vi "Temp Cluster Build.vi"() -> (8 "Bus":T1)   [LabVIEW 2011]
uses:
  Controls/1553_Bus.ctl
  Controls/1553_Bus_Controller.ctl
  Controls/1553_BC_Message.ctl
  Controls/1553 Param.ctl
  Controls/1553_Acyclic_Frame.ctl
  Controls/1553_Bus_Monitor.ctl
  Controls/1553_BM_Message.ctl
  Controls/1553_RT_Message.ctl
  AIT 1553 Custom Device.lvlib
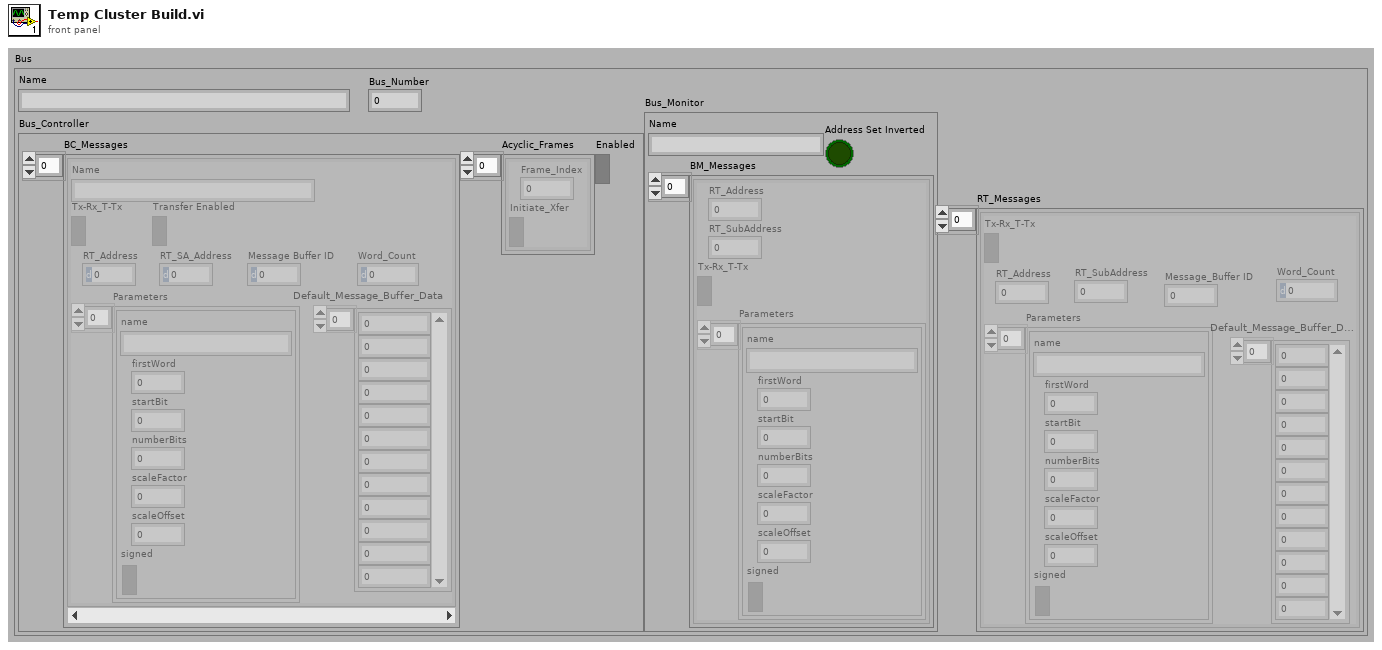
[diagram p1: front panel]
types:
  T1 = typedef "AIT 1553 Custom Device.lvlib/1553_Bus.ctl" = cluster{"Name":string, "Bus_Number":u8, "Bus_Controller":T2, "Bus_Monitor":T6, "RT_Messages":T8[]}
  T2 = typedef "AIT 1553 Custom Device.lvlib/1553_Bus_Controller.ctl" = cluster{"BC_Messages":T3[], "Acyclic_Frames":T5[], "Enabled":bool}
  T3 = typedef "AIT 1553 Custom Device.lvlib/1553_BC_Message.ctl" = cluster{"Name":string, "Tx-Rx_T-Tx":bool, "RT_Address":u8, "RT_SA_Address":u8, "Parameters":T4[], "Transfer Enabled":bool, "Message Buffer ID":u16, "Default_Message_Buffer_Data":u16[], "Word_Count":u8}
  T4 = typedef "AIT 1553 Custom Device.lvlib/1553 Param.ctl" = cluster{"name":string, "firstWord":i32, "startBit":i32, "numberBits":i32, "scaleFactor":dbl, "scaleOffset":dbl, "signed":bool}
  T5 = typedef "AIT 1553 Custom Device.lvlib/1553_Acyclic_Frame.ctl" = cluster{"Frame_Index":u8, "Initiate_Xfer":bool}
  T6 = typedef "AIT 1553 Custom Device.lvlib/1553_Bus_Monitor.ctl" = cluster{"Name":string, "BM_Messages":T7[], "Address Set Inverted":bool}
  T7 = typedef "AIT 1553 Custom Device.lvlib/1553_BM_Message.ctl" = cluster{"RT_Address":u8, "RT_SubAddress":u8, "Tx-Rx_T-Tx":bool, "Parameters":T4[]}
  T8 = typedef "AIT 1553 Custom Device.lvlib/1553_RT_Message.ctl" = cluster{"RT_Address":u8, "RT_SubAddress":u8, "Tx-Rx_T-Tx":bool, "Parameters":T4[], "Message_Buffer ID":u16, "Default_Message_Buffer_Data":u16[], "Word_Count":u8}
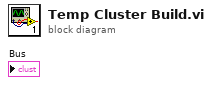
[diagram p0: block diagram]
diagram:
